vi "Generate Time Series (SubVI).vi"(5 "GY":dbl[][](array[numeric]), 7 "GX":dbl[][](array[numeric]), 8 "irData":i32[](array[numeric]), 10 "Start Index":i32, 11 "N Steps":i32) -> (3 "daqData":dbl[][](array[numeric]))   [LabVIEW 2020]
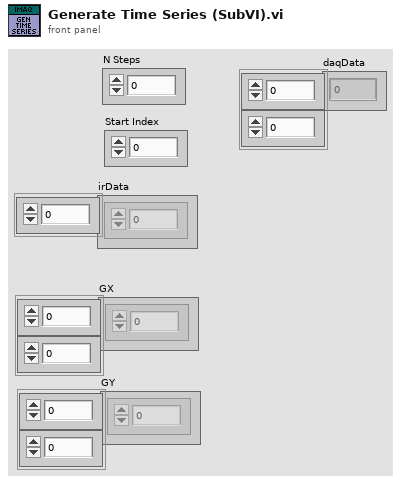
[diagram p1: front panel]
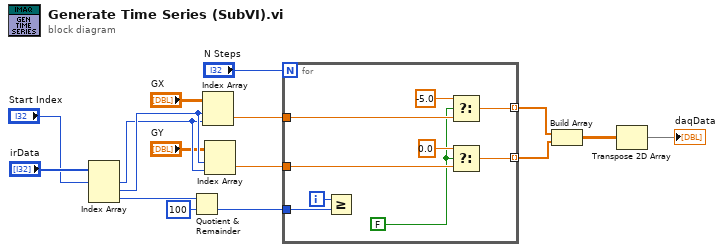
[diagram p0: block diagram]
diagram:
  n1 = Index Array(array="irData", index #1="Start Index") -> (element #1=w3:i32, element #2=w4:i32, element #3=w13:i32)  [unwired: 2 in]
  n2 = Quotient & Remainder(x=w13, y=100) -> (floor(x/y)=w12:i32)  [unwired: 1 out]
  n3 = Index Array(array="GX", index (row)=w4, index (col)=w3) -> (element=w5:dbl)
  n4 = Index Array(array="GY", index (row)=w4, index (col)=w3) -> (element=w1:dbl)
  n5 = for {
    N: "N Steps" -> [_]
    tunnel: w5 -> [w22]
    tunnel: w1 -> [w18]
    tunnel: [w25] -> w10 mode=indexing
    tunnel: w12 -> [w23]
    tunnel: [w19] -> w9 mode=indexing
    i -> [w24]
    w17 = FALSE ("x >= y?")
    n6 = Greater Or Equal?(x=w24, y=w23) -> ()  [unwired: 1 out]
    n7 = Select(t=-5.0, s=w17, f=w22) -> (s? t:f=w25:dbl)
    n8 = Select(t=0.0, s=w17, f=w18) -> (s? t:f=w19:dbl)
  }
  n9 = Build Array(w10, w9) -> (w8:dbl[][])
  n10 = Transpose 2D Array(2D array=w8) -> (transposed array=→"daqData":dbl[][])
